vi "Get Pixel Size.vi"(10 "ySize":sgl, 11 "xSize":sgl) -> (1 "function return":u32, 2 "ySize out":sgl, 3 "xSize out":sgl)   [LabVIEW 2018, in "Copy of Andor SDK.lvlib"]
doc: "EXPNETTYPE unsigned int WINAPI GetPixelSize(float * xSize, float * ySize);"
uses:
  Copy of Andor SDK.lvlib
  <userlib>/Andor SDK/ATMCD32D.dll
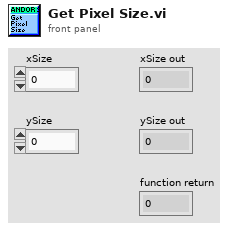
[diagram p1: front panel]
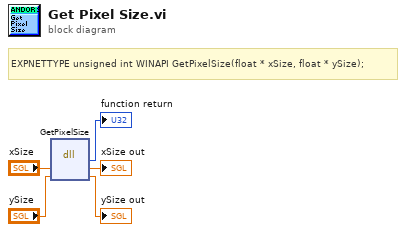
[diagram p0: block diagram]
diagram:
  # "EXPNETTYPE unsigned int WINAPI GetPixelSize(float * xSize, float * ySize);"
  n1 = dll-call lib="C:/Program Files (x86)/National Instruments/LabVIEW 2018/user.lib/Andor SDK/ATMCD32D.*" fn="GetPixelSize"("xSize"="xSize", "ySize"="ySize") -> (→"function return":u32, "xSize"=→"xSize out":sgl, "ySize"=→"ySize out":sgl)  [unwired: 3 in, 2 out]
